vi "RSZVB Set Coherent Signal Reference Port.vi"(8 "error in (no error)":errorcluster {"code" format="%.0x"}, 9 "Reference Port (1)":i32=1, 10 "Channel (1)":i32=1, 11 "VISA session":refnum<visa-resource-name>) -> (0 "error out":errorcluster {"code" format="%.0x"}, 3 "dup VISA session":refnum<visa-resource-name>)   [LabVIEW 2011]
doc: "This VI selects the reference port for the Defined Coherence Mode. \n\nNote(s):\n\n(1) This VI is not available for R&S ZVB instrument.\n\nRemote-control command(s):\nSOURce<Ch>:CMODe:RPORt"
uses:
  _utility/RSZVB Global Data.vi
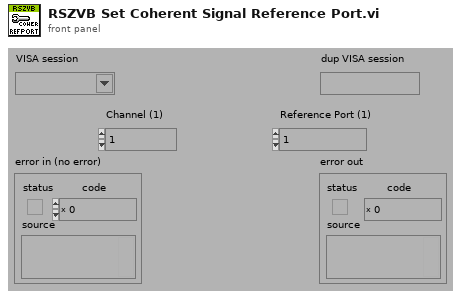
[diagram p1: front panel]
types:
  T1 = cluster{"Error Checking (T: On)":bool, "Installed Options":string[], "Data Valid?":bool, "Ports":i32, "Model":string[], "Option Checking (T: On)":bool}[]
  T2 = cluster{"Error Checking (T: On)":bool, "Installed Options":string[], "Data Valid?":bool, "Ports":i32, "Model":string[], "Option Checking (T: On)":bool}
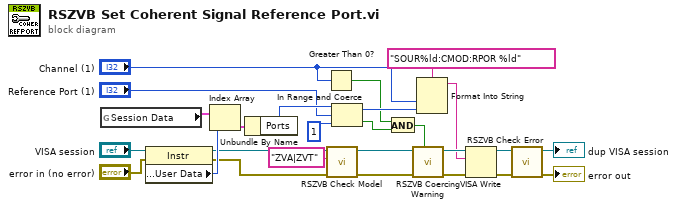
[diagram p0: block diagram]
diagram:
  n1 = global read "RSZVB Global Data.vi" "Session Data"() -> (w21:T1)
  n2 = property class="Instr"(reference="VISA session", error in="error in (no error)") -> (reference out=w2:refnum<visa-resource-name>, error out=w1:errorcluster, "General Settings:User Data"=w23:u32)
  n3 = Index Array(array=w21, index=w23) -> (element=w20:T2)
  n4 = Unbundle By Name(w20) -> ("Ports"=w24:i32)
  n5 = Greater Than 0?(x="Channel (1)") -> (x > 0?=w14:bool)
  n6 = call "RSZVB Check Model.vi"("error in (no error)"=w1, "Model"="ZVA|ZVT", "VISA session"=w2) -> ("error out"=w3:errorcluster, "dup VISA session"=w4:refnum<visa-resource-name>)  [unwired: 7 in]
  n7 = In Range and Coerce(upper limit=w24, x="Reference Port (1)", lower limit=1) -> (coerced(x)=w25:i32, In Range?=w15:bool)
  n8 = And(x=w14, y=w15) -> (x .and. y?=w26:bool)
  n9 = call "RSZVB Coercing Warning.vi"("In Range?"=w26, "error in (no error)"=w3, "VISA session"=w4) -> ("error out"=w17:errorcluster, "dup VISA session"=w18:refnum<visa-resource-name>)  [unwired: 7 in]
  n10 = Format Into String(format string="SOUR%ld:CMOD:RPOR %ld", "Channel (1)", w25) -> (resulting string=w16:string)  [unwired: 2 in, 1 out]
  n11 = VISA Write(VISA resource name=w18, write buffer=w16, error in (no error)=w17) -> (VISA resource name out=w9:refnum<visa-resource-name>, error out=w6:errorcluster)  [unwired: 1 out]
  n12 = call "RSZVB Check Error.vi"("error in (no error)"=w6, "VISA session"=w9) -> ("error out"=→"error out":errorcluster, "dup VISA session"=→"dup VISA session":refnum<visa-resource-name>)  [unwired: 8 in]
